vi "AssignColors.vi"(6 "Add Spaces?":bool, 11 "Code":refnum<vi>) -> (2 "Value":string)   [LabVIEW 2020]
uses:
  <vilib>/Utility/miscctls.llb/LVSelectionTypeDef.ctl
  ColorGlobals.vi
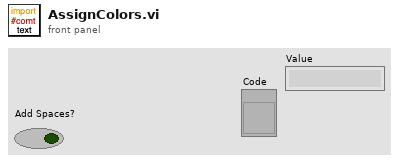
[diagram p1: front panel]
types:
  T1 = typedef "LVSelectionTypeDef.ctl" = cluster{"Selection Start":u32, "Selection End":u32}
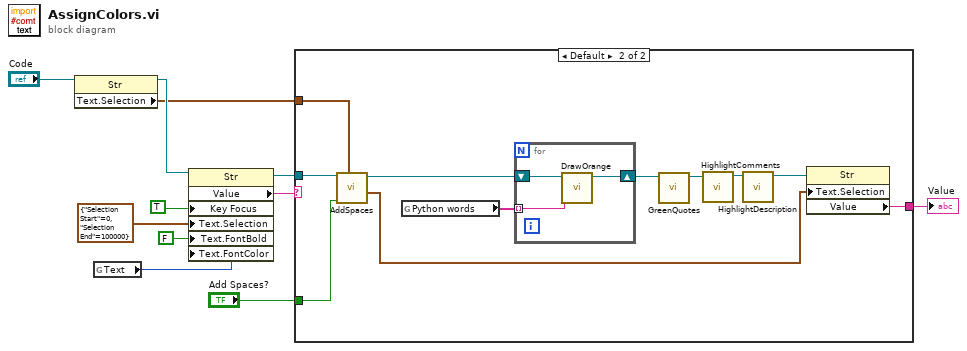
[diagram p0: block diagram]
diagram:
  n1 = property on="Property Node" class="Str"(reference="Code") -> (reference out=w8:refnum<vi>, "Text.Selection"=w7:T1)  [unwired: 1 in, 1 out]
  n2 = global read "ColorGlobals.vi" "Text"() -> (w1:u32)
  n3 = property on="Property Node" class="Str"(reference=w8, "Key Focus"=TRUE, "Text.Selection"=T1 {"Selection Start"=0, "Selection End"=100000}, "Text.FontBold"=FALSE ("Text.Font:Bold"), "Text.FontColor"=w1) -> (reference out=w3:refnum<vi>, "Value"=w2:string)  [unwired: 1 in, 1 out]
  n4 = case shown="Default" w2 {
    selector: w2 -> [w12 _]
    tunnel: w3 -> [_ w19]
    tunnel: w7 -> [_ w23]
    tunnel: [w12 w22] -> w5
    tunnel: "Add Spaces?" -> [_ w20]
    frame "" {
    }
    frame Default {
      n5 = call "AddSpaces.vi"("Text.Selection"=w23, "Add Spaces?"=w20, "String in"=w19) -> ("Cursor"=w21:cluster{u32, u32}, "String out"=w18:refnum<vi>)  [unwired: 7 in]
      n6 = global read "ColorGlobals.vi" "Python words"() -> (w13:string[])
      n7 = for {
        shift-right: [w25] -> w14
        shift-left: w18 -> [w26]
        tunnel: w13 -> [w24] mode=indexing
        n8 = call "DrawOrange.vi"("Expression"=w24, "String in"=w26) -> ("String out"=w25:refnum<vi>)  [unwired: 9 in]
      }
      n9 = call "GreenQuotes.vi"("String in"=w14) -> ("String out"=w15:refnum<vi>)  [unwired: 10 in]
      n10 = call "HighlightComments.vi"("String in"=w15) -> ("String out"=w16:refnum<vi>)  [unwired: 10 in]
      n11 = call "HighlightDescription.vi"("String in"=w16) -> ("String out"=w17:refnum<vi>)  [unwired: 10 in]
      n12 = property on="Property Node" class="Str"(reference=w17, "Text.Selection"=w21) -> ("Value"=w22:string)  [unwired: 1 in, 2 out]
    }
  }
  "Value" <- w5
